vi "get_magnet_value_from_MFT.vi"(10 "MFT name":string, 11 "isotope name":string) -> (3 "magnet value out":dbl)   [LabVIEW 2017]
doc: "uses the name of the MFT and the isotope name to retrieve the magnet value from the MFT"
uses:
  Classes/MagFieldTable/MagFieldTable.lvclass
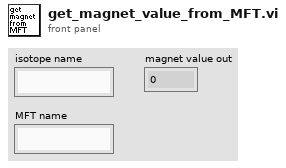
[diagram p1: front panel]
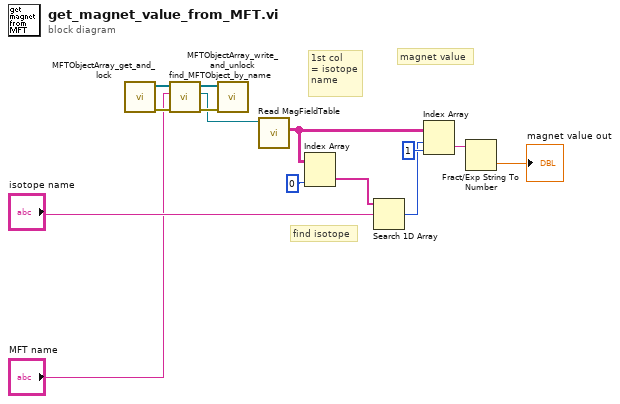
[diagram p0: block diagram]
diagram:
  # "magnet value"
  # "find isotope"
  # "1st col\n= isotope\nname"
  n1 = call "MFTObjectArray_get_and_lock.vi"() -> ("error out"=w6:errorcluster, "MFTObjects"=w1:refnum<class "MagFieldTable.lvclass">[])  [unwired: 10 in]
  n2 = call "find_MFTObject_by_name.vi"("error in (no error)"=w6, "MFT name"="MFT name", "MFTObjects in"=w1) -> ("error out"=w7:errorcluster, "found AnalyisObject"=w4:refnum<class "MagFieldTable.lvclass">, "MFTObjects out"=w2:refnum<class "MagFieldTable.lvclass">[])  [unwired: 5 in, 1 out]
  n3 = call "MFTObjectArray_write_and_unlock.vi"("error in (no error)"=w7, "MFTObjects"=w2) -> ()  [unwired: 9 in, 1 out]
  n4 = call-dynamic "Read MagFieldTable.vi"("MagFieldTable in"=w4) -> ("MagFieldTable"=w10:string[][])  [unwired: 8 in, 2 out]
  n5 = Index Array(array=w10, index (col)=0 ("disabled index (col)")) -> (element=w8:string[])  [unwired: 1 in]
  n6 = Search 1D Array(1D array=w8, element="isotope name") -> (index of element=w11:i32)  [unwired: 1 in]
  n7 = Index Array(array=w10, index (row)=w11, index (col)=1 ("disabled index (col)")) -> (element=w13:string)
  n8 = Fract/Exp String To Number(string=w13) -> (number=→"magnet value out":dbl)  [unwired: 3 in, 1 out]
